vi "NodeElmWidth.vi"() -> ()   [LabVIEW 2017, in "XDataNode.xnode"]
uses:
  <vilib>/Platform/TimedLoop/XDataNode/XDataNode.xnode
panel:
  in  "Node Element width":u32=15
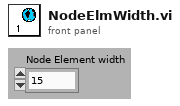
[diagram p1: front panel]
diagram:
